vi "Motor-Move-Rel-bwait.vi"(1 "bWait":bool, 3 "error":errorcluster, 4 "Posição":sgl, 5 "MG17Motor A":refnum<k7>) -> (0 "error out":errorcluster, 2 "MG17Motor out":refnum<k7>)   [LabVIEW 2021]
doc: "André Romero - 2016\nandretec@ifsc.usp.br\nIFSC - USP"
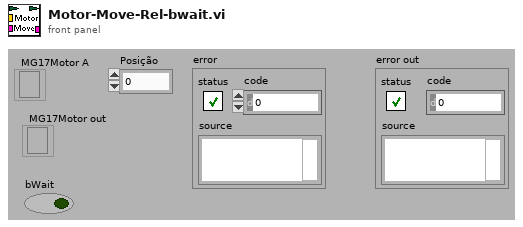
[diagram p1: front panel]
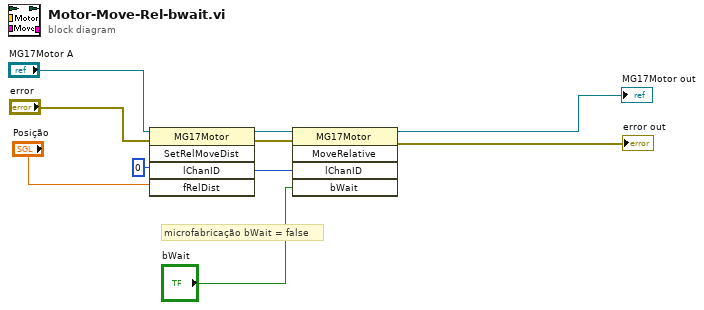
[diagram p0: block diagram]
diagram:
  # "microfabricação bWait = false"
  n1 = invoke class="MG17Motor" method="SetRelMoveDist"(reference="MG17Motor A", error in="error", "lChanID"=0, "fRelDist"="Posição") -> (reference out=w6:refnum<k7>, error out=w9:errorcluster, "lChanID"=w10:i32)  [unwired: 1 in, 2 out]
  n2 = invoke class="MG17Motor" method="MoveRelative"(reference=w6, error in=w9, "lChanID"=w10, "bWait"="bWait") -> (reference out=→"MG17Motor out":refnum<k7>, error out=→"error out":errorcluster)  [unwired: 1 in, 3 out]
